vi "GT Compare Linear.vi"(0 "cardNum":i16, 1 "repeatTimes":i32, 2 "time":i16, 5 "encoder":i16, 7 "channel":i16, 9 "startPos":i32, 11 "error in (no error)":errorcluster caption="错误输入（无错误）", 12 "interval":i32, 13 "source":i16) -> (4 "function return":i16, 15 "error out":errorcluster caption="错误输出")   [LabVIEW 2014, in "gts.lvlib"]
doc: "GT_API GT_CompareLinear(short cardNum,short encoder,short channel,long startPos,long repeatTimes,long interval,short time,short source);"
uses:
  gts.lvlib
  gts.dll
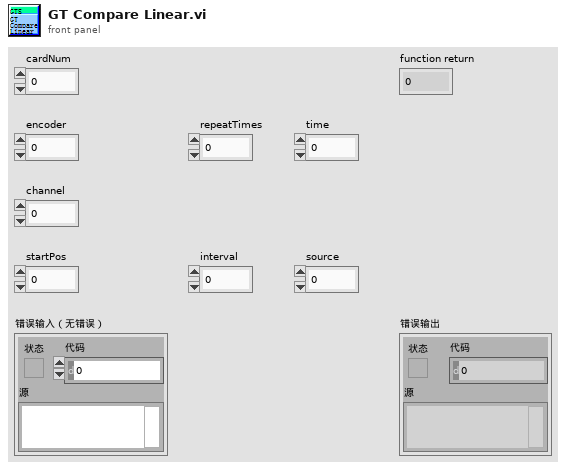
[diagram p1: front panel]
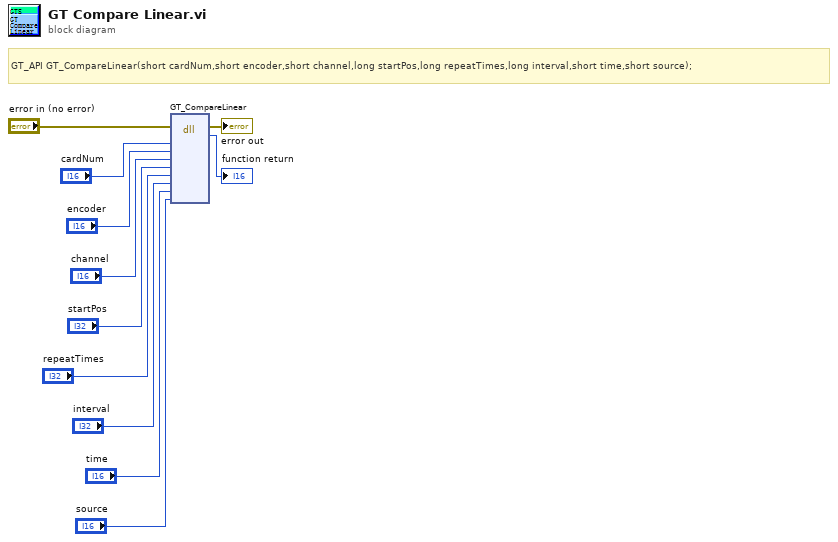
[diagram p0: block diagram]
diagram:
  # "GT_API GT_CompareLinear(short cardNum,short encoder,short channel,long startPos,long repeatTimes,long interval,short time,short source);"
  n1 = dll-call lib="PTH2?abs D\t王淼清$控制卡常用功能例程(Labview)gts.*" fn="GT_CompareLinear"(error in="error in (no error)", "cardNum"="cardNum", "encoder"="encoder", "channel"="channel", "startPos"="startPos", "repeatTimes"="repeatTimes", "interval"="interval", "time"="time", "source"="source") -> (error out=→"error out":errorcluster, →"function return":i16)  [unwired: 10 in, 1 out]
